vi "router.vi"() -> ()   [LabVIEW 2012]
uses:
  <vilib>/addons/zeromq/socket_type.ctl
  <vilib>/addons/zeromq/socket_options.ctl
  <vilib>/addons/zeromq/zeromq.lvlib
panel:
  in  "Volume":i32=40000
  out "error out":errorcluster
  in  "정지":bool
  in  "endpoint":string="tcp://127.0.0.1:5557"
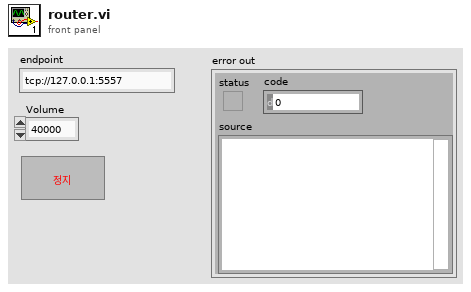
[diagram p1: front panel]
types:
  T1 = typedef "zeromq.lvlib/socket_options.ctl" = enum8{"NONE", "ZMQ_HWM", "<2>", "ZMQ_SWAP", "ZMQ_AFFINITY", "ZMQ_IDENTITY", "ZMQ_SUBSCRIBE", "ZMQ_UNSUBSCRIBE", "ZMQ_RATE", "ZMQ_RECOVERY_IVL", "ZMQ_MCAST_LOOP", "ZMQ_SNDBUF", "ZMQ_RCVBUF", "ZMQ_RCVMORE", "ZMQ_FD", "ZMQ_EVENTS", "ZMQ_TYPE", "ZMQ_LINGER", "ZMQ_RECONNECT_IVL", "ZMQ_BACKLOG", "ZMQ_RECOVERY_IVL_MSEC", "ZMQ_RECONNECT_IVL_MAX", "ZMQ_MAXMSGSIZE", "ZMQ_SNDHWM", "ZMQ_RCVHWM", "ZMQ_MULTICAST_HOPS", "<26>", "ZMQ_RCVTIMEO", "ZMQ_SNDTIMEO", "<29>", "<30>", "ZMQ_IPV4ONLY", "ZMQ_LAST_ENDPOINT", "ZMQ_ROUTER_MANDATORY", "ZMQ_TCP_KEEPALIVE", "ZMQ_TCP_KEEPALIVE_CNT", "ZMQ_TCP_KEEPALIVE_IDLE", "ZMQ_TCP_KEEPALIVE_INTVL", "ZMQ_TCP_ACCEPT_FILTER", "ZMQ_DELAY_ATTACH_ON_CONNECT", "ZMQ_XPUB_VERBOSE"}
  T2 = typedef "zeromq.lvlib/socket_type.ctl" = enum8{"ZMQ_PAIR", "ZMQ_PUB", "ZMQ_SUB", "ZMQ_REQ", "ZMQ_REP", "ZMQ_DEALER", "ZMQ_ROUTER", "ZMQ_PULL", "ZMQ_PUSH", "ZMQ_XPUB", "ZMQ_XSUB"}
  T3 = typedef "pointer.ctl" = u64
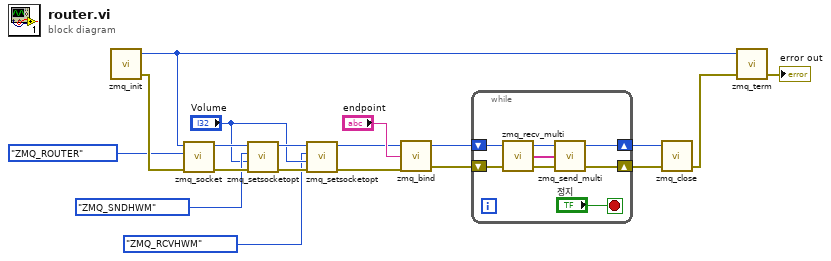
[diagram p0: block diagram]
diagram:
  n1 = call <vilib>:"zmq_init.vi"() -> ("error out"=w19:errorcluster, "context"=w11:T3)  [unwired: 4 in]
  n2 = call <vilib>:"zmq_socket.vi"("error in"=w19, "socket type"=socket_type."ZMQ_ROUTER", "ctx in"=w11) -> ("error out"=w8:errorcluster, "socket"=w9:T3)  [unwired: 3 in]
  n3 = call <vilib>:"zmq_setsocketopt.vi"("error in"=w8, "value"="Volume", "option"=socket_options."ZMQ_SNDHWM", "socket in"=w9) -> ("error out"=w4:errorcluster, "socket out"=w6:T3)  [unwired: 2 in]
  n4 = call <vilib>:"zmq_setsocketopt.vi"("error in"=w4, "value"="Volume", "option"=socket_options."ZMQ_RCVHWM", "socket in"=w6) -> ("error out"=w3:errorcluster, "socket out"=w5:T3)  [unwired: 2 in]
  n5 = call <vilib>:"zmq_bind.vi"("error in"=w3, "endpoint"="endpoint", "socket in"=w5) -> ("error out"=w15:errorcluster, "socket out"=w16:T3)  [unwired: 1 in]
  n6 = while {
    shift-right: [w22] -> w13
    shift-left: w16 -> [w26]
    shift-right: [w21] -> w14
    shift-left: w15 -> [w27]
    stop <- "정지" stop-if-true
    n7 = call <vilib>:"zmq_recv_multi.vi"("error in"=w27, "socket in"=w26) -> ("error out"=w25:errorcluster, "parts"=w24:string[], "socket out"=w23:T3)  [unwired: 1 in]
    n8 = call <vilib>:"zmq_send_multi.vi"("error in"=w25, "parts"=w24, "socket in"=w23) -> ("error out"=w21:errorcluster, "socket out"=w22:T3)  [unwired: 1 in]
  }
  n9 = call <vilib>:"zmq_close.vi"("error in"=w14, "socket in"=w13) -> ("error out"=w12:errorcluster)  [unwired: 3 in]
  n10 = call <vilib>:"zmq_term.vi"("error in"=w12, "context"=w11) -> ("error out"=→"error out":errorcluster)  [unwired: 3 in]
